vi "Drive Encoder Counter.vi"   [LabVIEW 2009]
uses:
  Motor Encoder Global.vi
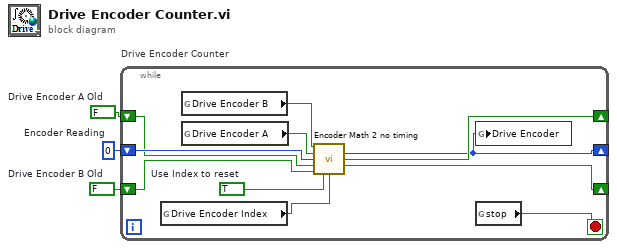
[diagram p0: block diagram]
diagram:
  w3 = 0  # Encoder Reading
  w2 = FALSE  # Drive Encoder A Old
  w1 = FALSE  # Drive Encoder B Old
  n1 = while "Drive Encoder Counter" {
    shift-right: [w13] -> _
    shift-left: w2 -> [w12]
    shift-right: [w11] -> _
    shift-left: w1 -> [w10]
    shift-right: [w5] -> _
    shift-left: w3 -> [w14]
    stop <- w9 stop-if-true
    w4 = TRUE  # Use Index to reset
    n2 = global read "Motor Encoder Global.vi" "Drive Encoder Index"() -> (w6:bool)
    n3 = global read "Motor Encoder Global.vi" "Drive Encoder B"() -> (w8:bool)
    n4 = global read "Motor Encoder Global.vi" "Drive Encoder A"() -> (w7:bool)
    n5 = call "Encoder Math 2 no timing.vi"("Encoder B"=w8, "Encoder A"=w7, "Encoder Reading"=w14, "Encoder A Old"=w12, "Encoder B Old"=w10, "Use Index to reset"=w4, "Encoder Index"=w6) -> ("Count Zeroed at Index"=w5:i32, "Encoder A Old (sReg)"=w13:bool, "Encoder B Old (sReg)"=w11:bool)  [unwired: 3 in, 3 out]
    n6 = global write "Motor Encoder Global.vi" "Drive Encoder"(w5) -> ()
    n7 = global read "Motor Encoder Global.vi" "stop"() -> (w9:bool)
  }
